vi "tableau.vi"() -> ()   [LabVIEW 2014]
panel:
  out "nbr lement":i32
  out "Multiplication":dbl
  out "somme":dbl
  in  "Array":dbl[](array[numeric])
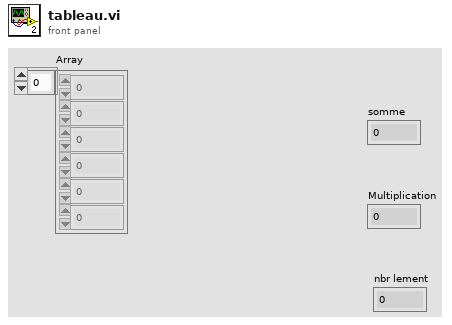
[diagram p1: front panel]
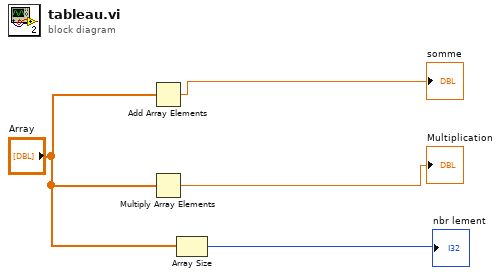
[diagram p0: block diagram]
diagram:
  n1 = Add Array Elements(numeric array="Array") -> (sum=→"somme":dbl)
  n2 = Multiply Array Elements(1:"Array") -> (0:→"Multiplication":dbl)
  n3 = Array Size(array="Array") -> (size(s)=→"nbr lement":i32)
